vi "ni579x Construct Command Set LO Frequency.vi"(0 "Register Bus":refnum<class "ni579x Register Bus v1 Host.lvclass">=refnum, 1 "scope":string, 5 "frequency [Hz]":dbl format="%#_6p", 11 "Error In":errorcluster) -> (4 "Register Bus (out)":refnum<class "ni579x Register Bus v1 Host.lvclass">, 6 "FAM Register Operations":T1[](array[typedef]) {"Write Data" format="%x"; "Address" format="%06x"; "FAM Register Offset" items=["ADC"=1, "DAC"=2, "Clock Distribution Chip"=3, "Frequency/Phase Adjust DAC"=4, "EEPROM"=5, "EEPROM Commands"=6, "LO1"=7, "Rx Atten Pre-LNA"=9, "Rx Atten Post-LNA"=10, "Tx Atten"=11]}, 10 "coerced frequency [Hz]":dbl format="%#_6p", 15 "Error Out":errorcluster)   [LabVIEW 2013]
uses:
  <instrlib>/ni579x/Register Bus/v1/Host/ni579x Register Bus v1 Host.lvclass
  <instrlib>/ni579x/Config/v1/Shared/Types/ni579x FAM Register Operation.ctl
  <instrlib>/ni579x/Config/v1/Shared/Types/ni579x FAM Register Offset.ctl
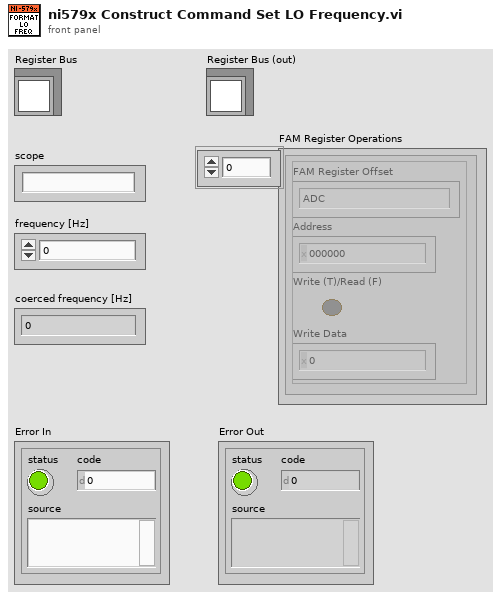
[diagram p1: front panel]
types:
  T1 = typedef "ni579x FAM Register Operation.ctl" = cluster{"FAM Register Offset":T2, "Address":u32, "Write (T)/Read (F)":bool, "Write Data":u32}
  T2 = typedef "ni579x FAM Register Offset.ctl" = u8
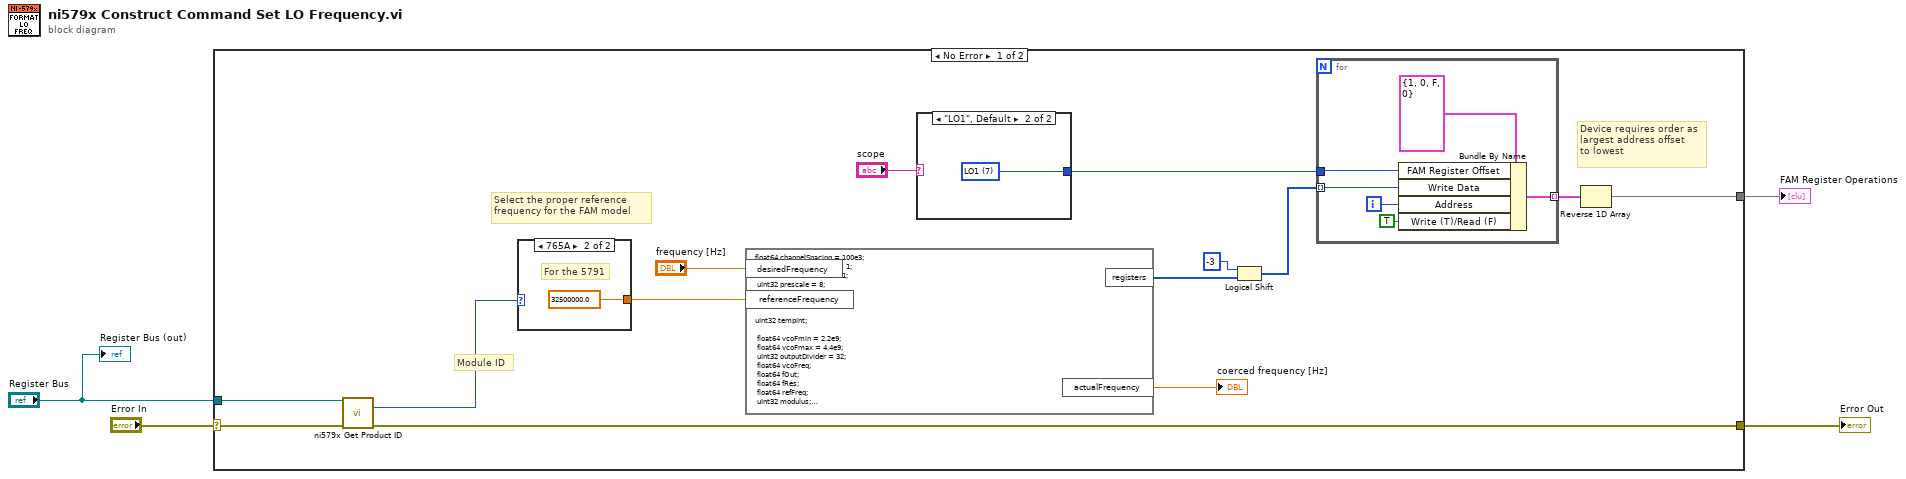
[diagram p0: block diagram]
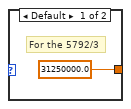
[diagram p2: hidden frame]
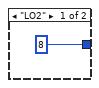
[diagram p3: hidden frame]
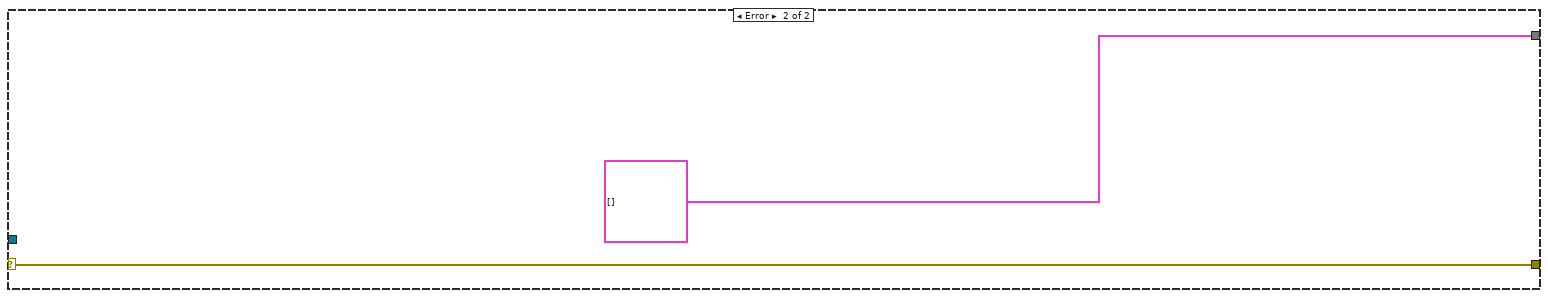
[diagram p4: hidden frame]
diagram:
  n1 = case shown="No Error" "Error In" {
    selector: "Error In" -> [w8 w30]
    tunnel: [w7 w30] -> w3
    tunnel: "Register Bus" -> [w6 _]
    tunnel: [w11 T1[] [] ("SPI Instructions")] -> w1
    frame No Error {
      # "Module ID"
      # "Select the proper reference \nfrequency for the FAM model"
      # "Device requires order as\nlargest address offset\nto lowest"
      n2 = call <instrlib>:"ni579x Get Product ID.vi"("Register Bus"=w6, "Error In"=w8) -> ("product ID"=w5:u16, "Error Out"=w7:errorcluster)  [unwired: 11 in, 1 out]
      n3 = case shown="765A" w5 {
        tunnel: [31250000.0 ("input variable") 32500000.0 ("input variable")] -> w9
        frame Default {
          # "For the 5792/3"
        }
        frame 30298 {
          # "For the 5791"
        }
      }
      n4 = formula code="float64 channelSpacing = 100e3;\n\tuInt32 referenceDivider = 1;\n\tint referencePrescale = -1;\n\tuInt32 prescale = 8;\n\nuInt32 refPrescaleBits;\n\nuInt32 tempInt;\n\n\tfloat64 vcoFmin = 2.2e9;\n\tfloat64 vcoFmax = 4.4e9;\n\tuInt32 outputDivider = 32;\n\tfloat64 vcoFreq;\n\tfloat64 fOut;\n\tfloat64 fRes;\n\tfloat64 refFreq;\n\tuInt32 modulus;\n\tuInt32 clkDiv;\n\tuInt32 integer;\n\tuInt32 frac;\n\tuInt32 phase = 1;\n\tuInt32 lsm = 0;\n\tuInt32 muxOut = 0;\n\tuInt32 lockDetect = 1;\n\n\tuInt32 vRef = 0;\t\n\tuInt32 csr = 0;\n\tuInt32 phaseReSync = 0;\n\tuInt32 fastLock = 0;\n\tuInt32 flcClkDiv = 150;\n\n\tuInt32 output = 3;\n\tuInt32 outputEnabled = 1;\n\tuInt32 aux = 0;\n\tuInt32 auxEnabled = 0;\n\tuInt32 vcoPdu = 0;\n\tuInt32 mtld = 0;\n\tuInt32 auxOutSel = 0;\n\tuInt32 feedbackSelect = 1;\n\n\tuInt32 doubleBuffer = 0;\n\tuInt32 icp = 7;\n\tuInt32 ldf = 0;\n\tuInt32 ldp = 0;\n\tuInt32 pdPolarity = 1;\n\tuInt32 powerDown = 0;\n\tuInt32 cpThreeState = 0;\n\tuInt32 counterReset = 0;\n\n\tuInt32 registers[6];\n\n\tfloat64 x[101];\n\tfloat64 nu[101];\n\tfloat64 de[101];\n\tfloat64 c[101];\n\tint trash;\n\tint i;\n\nfloat64 fpd;\nfloat64 actualFrequency;\n\n\tif(referencePrescale == -1){\n\trefPrescaleBits = 1;\nrefFreq = referenceFrequency * (0.5 / referenceDivider);\n}\telse if(referencePrescale == 0){\n\trefPrescaleBits = 0;\nrefFreq = referenceFrequency * (1.0 / referenceDivider);\n}else if(referencePrescale == 1){\n\trefPrescaleBits = 2;\nrefFreq = referenceFrequency * (2.0 / referenceDivider);\n}\n\t\n\t// calculate the actual output frequency\n\tfOut = floor(desiredFrequency / channelSpacing + 0.5) * channelSpacing;\n//\tif(fOut < 137.5e6 || fOut > 4.4e9) return 1;\n\t\n\t// calculate the output divider\n\tdo{\n\t\toutputDivider >>= 1;\n\t\tvcoFreq = fOut * outputDivider;\n\t} while(vcoFreq > vcoFmax);\n\n\tfRes = channelSpacing * outputDivider;\n\tclkDiv = floor(8 * refFreq / 1.0e6 + 0.5);\n\tmodulus = floor(refFreq / fRes + 0.5);\n\tinteger = floor(vcoFreq / refFreq);\n\tif(integer > 65535) integer = 65535;\n\tif(integer < 23) integer = 23;\n\tif(prescale == 8)\n\t\tif(integer < 75) integer = 75;\n\n\n\ttrash = 0;\n\n\tc[0] = vcoFreq / refFreq - integer;\n\n\tif(abs(c[0]) > 0.0001) {\n\t\tdo{\n\t\t\ttrash++;\n\t\t\tx[trash] = floor(1.0 / c[trash - 1]);\n\t\t\tc[trash] = 1.0 / c[trash - 1] - x[trash];\n\t\t} while( (abs(c[trash]) >= 0.001) && (trash < 98));\n\t\tnu[trash] = 1.0;\n\t\tde[trash] = x[trash];\n\t\twhile(trash > 1){\n\t\t\ttrash--;\n\t\t\tnu[trash] = de[trash + 1];\n   tempInt = de[trash + 1] * x[trash] + nu[trash + 1];\n\t\t\tde[trash] = tempInt & 4095;\n\t\t}\n\t\tmodulus = de[1];\n\t} else {\n\t\tmodulus = (refFreq / fRes);\n\t}\n\n\tif(modulus < 2) modulus = 2;\n\tif(modulus > 4095) modulus = 4095;\n\tfrac =  floor(modulus * (vcoFreq / refFreq - integer) + 0.5);\n\tif(frac < 0) frac = 0;\n\tif(frac > 4095) frac = 4095;\n\tif(frac >= modulus){\n\t\tinteger += (frac / modulus);\n\t\tfrac -= (modulus * (frac / modulus));\n\t}\n\n\tregisters[0] = ((integer << 12) + frac) << 3;\n\tregisters[1] = ((((prescale - 4) << 22) + (phase << 12) + modulus) << 3) + 1;\n\tregisters[2] = ((((lsm * 3) << 26) +(muxOut << 23) + (refPrescaleBits << 21) + (referenceDivider << 11) + (doubleBuffer << 10) + (icp << 6)+ (ldf << 5) + (ldp << 4) + (pdPolarity << 3) + (powerDown << 2) + (cpThreeState << 1) + counterReset) << 3) + 2;\n\tregisters[3] = (((vRef << 16) +(csr << 15) + (phaseReSync << 13) + (fastLock << 12) + flcClkDiv) << 3) + 3;\n tempInt = log(outputDivider) / log(2);\n\tregisters[4] = ((output + (outputEnabled << 2) + (aux << 3) + (auxEnabled << 5) + (clkDiv << 9) + (vcoPdu << 8) + (mtld << 7) + (auxOutSel << 6) + (tempInt << 17) + (feedbackSelect << 20)) << 3) + 4;\n\tregisters[5] = (((1 << 16) + (1 << 17) + (lockDetect << 19)) << 3) + 5;\n\nfpd = refFreq / referenceDivider;\nactualFrequency = (integer + frac / modulus) * fpd / outputDivider;"("desiredFrequency"="frequency [Hz]", "referenceFrequency"=w9) -> ("registers"=w14:u32[], "actualFrequency"=→"coerced frequency [Hz]":dbl)
      n5 = case shown="\"LO1\", Default" "scope" {
        tunnel: [u8 8 w22] -> w12
        frame "LO2" {
        }
        frame "LO1", Default {
          w22 = T2 7 items=["ADC"=1, "DAC"=2, "Clock Distribution Chip"=3, "Frequency/Phase Adjust DAC"=4, "EEPROM"=5, "EEPROM Commands"=6, "LO1"=7, "Rx Atten Pre-LNA"=9, "Rx Atten Post-LNA"=10, "Tx Atten"=11] ("FAM Register Offset")
        }
      }
      n6 = Logical Shift(y=i8 -3, x=w14) -> (x << y=w17:u32[])
      n7 = for {
        tunnel: w17 -> [w28] mode=indexing
        tunnel: [w26] -> w16 mode=indexing
        tunnel: w12 -> [w25]
        i -> [w27]
        n8 = Bundle By Name(cluster=T1 {"FAM Register Offset"=1, "Address"=0, "Write (T)/Read (F)"=FALSE, "Write Data"=0} ("FAM Register Operation"), "FAM Register Offset"=w25, "Write Data"=w28, "Address"=w27, "Write (T)/Read (F)"=TRUE) -> (w26:T1)
      }
      n9 = Reverse 1D Array(array=w16) -> (reversed array=w11:T1[])
    }
    frame Error {
    }
  }
  "Error Out" <- w3
  "FAM Register Operations" <- w1
  "Register Bus (out)" <- "Register Bus"
